vi "Remove Tags.vi"(9 "separators":string[](array[string]), 11 "String in":string) -> (1 "array size":i32, 2 "index array":i32[][](array[numeric]), 3 "String out":string)   [LabVIEW 2017]
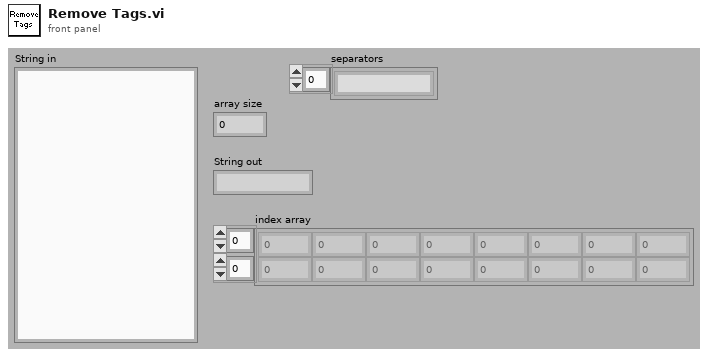
[diagram p1: front panel]
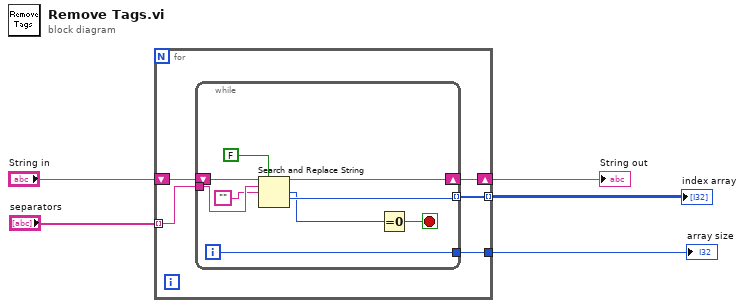
[diagram p0: block diagram]
diagram:
  n1 = for {
    tunnel: "separators" -> [w10] mode=indexing
    shift-right: [w9] -> w4
    shift-left: "String in" -> [w8]
    tunnel: [w7] -> w2 mode=indexing
    tunnel: [w6] -> w3
    n2 = while {
      tunnel: w10 -> [w18]
      tunnel: [w15] -> w7 mode=indexing
      shift-right: [w16] -> w9
      shift-left: w8 -> [w12]
      tunnel: [w11] -> w6
      i -> [w11]
      stop <- w13 stop-if-true
      n3 = Search and Replace String(replace all?=FALSE ("replace all? (F)"), input string=w12, search string=w18, replace string="") -> (result string=w16:string, number of replacements=w14:i32, offset past replacement=w15:i32)  [unwired: 1 in, 4 out]
      n4 = Equal To 0?(x=w14) -> (x = 0?=w13:bool)
    }
  }
  "String out" <- w4
  "array size" <- w3
  "index array" <- w2
